vi "add_timedelay_exp.vi"(2 "error in (no error)":errorcluster, 3 "delay":dbl, 4 "Experiment.lvclass in":refnum<class "Experiment.lvclass">) -> (0 "error out":errorcluster, 1 "Experiment.lvclass out":refnum<class "Experiment.lvclass">)   [LabVIEW 2018, in "Experiment.lvclass"]
uses:
  Experiment.lvclass
  Experiment.lvclass/Experiment.ctl
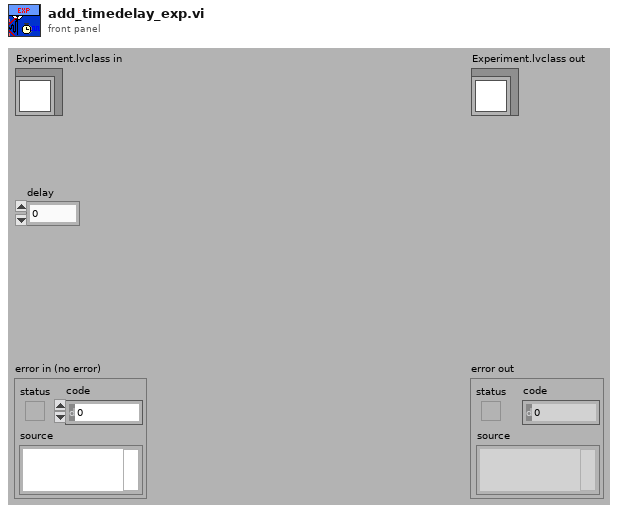
[diagram p1: front panel]
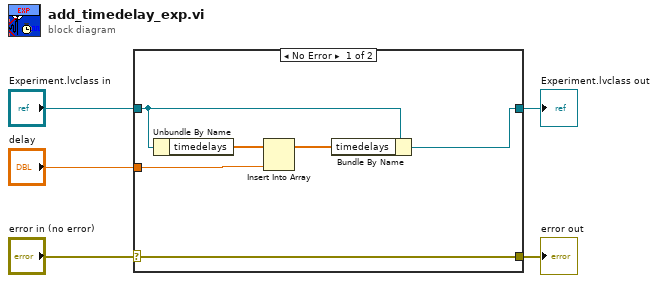
[diagram p0: block diagram]
diagram:
  n1 = case shown="No Error" "error in (no error)" {
    selector: "error in (no error)" -> [w11 w12]
    tunnel: [w11 w12] -> w4
    tunnel: [w10 w13] -> w2
    tunnel: "Experiment.lvclass in" -> [w9 w13]
    tunnel: "delay" -> [w6 _]
    frame No Error {
      n2 = Unbundle By Name(w9) -> ("timedelays"=w8:dbl[])
      n3 = Insert Into Array(array=w8, new element=w6) -> (w7:dbl[])  [unwired: 1 in]
      n4 = Bundle By Name(cluster=w9, "timedelays"=w7) -> (w10:refnum<class "Experiment.lvclass">)
    }
    frame Error {
    }
  }
  "error out" <- w4
  "Experiment.lvclass out" <- w2
